vi "Stream_lock_in_data.vi"(4 "Input signal 2":dbl[][](graph)=[[-0.008779764175415039, -0.004544258117675781, 0.001982450485229492, 0.0061130523681640625, 0.012277364730834961, 0.02335667610168457, 0.03196120262145996, 0.03911137580871582, 0.046051740646362305, 0.054459571838378906, 0.056176185607910156, 0.06710648536682129, 0.06688714027404785, 0.0721597671508789, 0.0703728199005127, 0.06852388381958008, 0.05539417266845703, 0.05409598350524902, 0.04247546195983887, 0.037828683853149414, 0.029506683349609375, 0.02313971519470215, 0.011553764343261719, 0.008774995803833008, -0.00023245811462402344, -0.007607936859130859, -0.013626813888549805, -0.021468400955200195, -0.02878427505493164, -0.03249406814575195, -0.04259824752807617, -0.054628849029541016, -0.06337881088256836, -0.07187247276306152, -0.07883429527282715, -0.07958292961120605, -0.08783698081970215, -0.0936126708984375, -0.09322285652160645, -0.09287834167480469, -0.08769989013671875, -0.08086681365966797, -0.07571101188659668, -0.07127642631530762, -0.05929231643676758, -0.0570833683013916, -0.043621063232421875, -0.03627181053161621, -0.0225830078125, -0.019170045852661133], [0.0009274482727050781, 0.007216930389404297, 0.009523630142211914, 0.016843080520629883, 0.01917123794555664, 0.014799833297729492, 0.016978979110717773, 0.02221822738647461, 0.028494596481323242, 0.030884742736816406, 0.0387883186340332, 0.03027796745300293, 0.036940574645996094, 0.029010772705078125, 0.030074119567871094, 0.027055740356445312, 0.03615736961364746, 0.025472640991210938, 0.02970099449157715, 0.017670392990112305, 0.013712644577026367, 0.007717609405517578, 0.011627674102783203, 0.000896453857421875, 0.004842281341552734, 0.00044226646423339844, -0.0009751319885253906, -0.0026845932006835938, -0.004961490631103516, -0.014774799346923828, -0.010123252868652344, -0.00890493392944336, -0.009294748306274414, -0.011196136474609375, -0.013052225112915039, -0.02232074737548828, -0.016134977340698242, -0.01260995864868164, -0.012656450271606445, -0.011260509490966797, -0.014526844024658203, -0.017745494842529297, -0.012099742889404297, -0.007849931716918945, -0.00917673110961914, 0.004441738128662109, -0.0028061866760253906, 0.001468658447265625, -0.005977153778076172, 0.0028574466705322266], [0.08533358573913574, 0.10965466499328613, 0.1100766658782959, 0.143967866897583, 0.15009522438049316, 0.15192270278930664, 0.138627290725708, 0.14617443084716797, 0.14183402061462402, 0.15452861785888672, 0.15473365783691406, 0.1419377326965332, 0.13108372688293457, 0.11727333068847656, 0.11010408401489258, 0.11058330535888672, 0.11924505233764648, 0.09971499443054199, 0.08461117744445801, 0.047779083251953125, 0.029468536376953125, 0.01607537269592285, 0.02023935317993164, -0.008087158203125, -0.020216703414916992, -0.04974365234375, -0.05224108695983887, -0.05714774131774902, -0.04624128341674805, -0.06816744804382324, -0.07148623466491699, -0.09539961814880371, -0.09099602699279785, -0.09783506393432617, -0.08560299873352051, -0.10595440864562988, -0.0937807559967041, -0.10118484497070312, -0.08174419403076172, -0.07831931114196777, -0.05225181579589844, -0.05335092544555664, -0.026574134826660156, -0.016901493072509766, 0.007963180541992188, 0.03178834915161133, 0.042150020599365234, 0.04857063293457031, 0.05016446113586426, 0.06906867027282715]], 5 "decimating factor":i32=400, 6 "Field":dbl=-90000.125 format="%#_10f", 7 "Temperature":dbl=0.049972 format="%#_10f", 8 "Time":dbl=8433065.97 format="%#_10f") -> ()   [LabVIEW 2013]
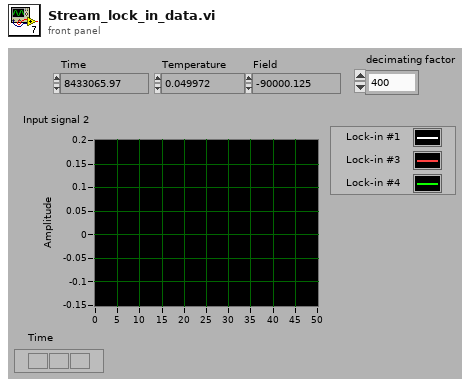
[diagram p1: front panel]
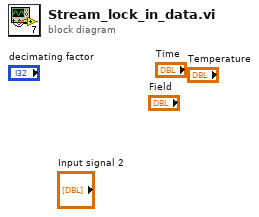
[diagram p0: block diagram]
diagram:
